vi "Read Pixels.vi"(8 "error in (no error)":errorcluster, 10 "Rectangle":T1={"x"=0, "y"=0, "Width"=1000, "Height"=1000}, 11 "Renderer":refnum<class "Renderer.lvclass">) -> (0 "error out":errorcluster, 3 "Pixels":i32[][](array[numeric]))   [LabVIEW 2021, in "Renderer.lvclass"]
uses:
  Renderer.lvclass
  Renderer.lvclass/Renderer.ctl
  LabSDL2/Source/Libraries/LibSDL2 Wrapper/LibSDL2.lvlib
  LabSDL2/Source/Libraries/LibSDL2 Wrapper/Controls/Rectangle.ctl
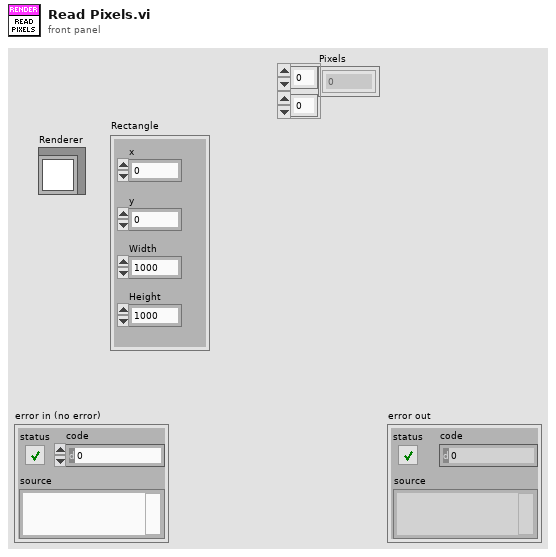
[diagram p1: front panel]
types:
  T1 = typedef "LibSDL2.lvlib/Rectangle.ctl" = cluster{"x":i32, "y":i32, "Width":i32, "Height":i32}
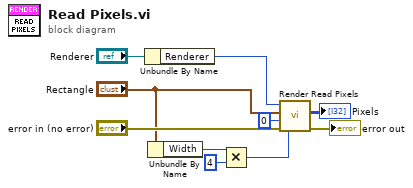
[diagram p0: block diagram]
diagram:
  n1 = Unbundle By Name("Renderer") -> ("Renderer"=w7:u32)
  n2 = Unbundle By Name("Rectangle") -> ("Width"=w4:i32)
  n3 = Multiply(x=w4, y=4) -> (x*y=w2:i32)
  n4 = call "Render Read Pixels.vi"("Pitch"=w2, "error in"="error in (no error)", "Format"=u32 0, "Rectangle"="Rectangle", "Renderer Pointer"=w7) -> ("error out"=→"error out":errorcluster, "Pixels"=→"Pixels":i32[][])  [unwired: 4 in, 1 out]
